vi "Front Panel Clean-Up.vi"(6 "Variant in":variant, 7 "Shift Pressed?":bool, 8 "error in (no error)":errorcluster, 10 "QD Combo Box Ref":refnum<vi>, 11 "QD Launch VI Ref":refnum<vi>) -> (0 "error out":errorcluster, 4 "Variant out":variant)   [LabVIEW 2011, in "LVH-Toolbox.lvlib"]
doc: "Write a 1-2 sentence description of the functionality of your plugin here. Replace the \"$\" below with the character you wish to assign as the default shortcut for this plugin. Do not add any text after the 'Default Shortcut' line below.\n\nDefault Shortcut - [$]"
uses:
  <vilib>/LabVIEW Hacker/LVH-Toolbox/LVH-Toolbox.lvlib
panel:
  in  "Undo Name":string="Quick Drop Front Panel Clean-Up"
  # "Do not change the connector pane of this VI.\n\nSee the block diagram for directions on how to use this template."
  # "Specify the name of the Undo transaction"
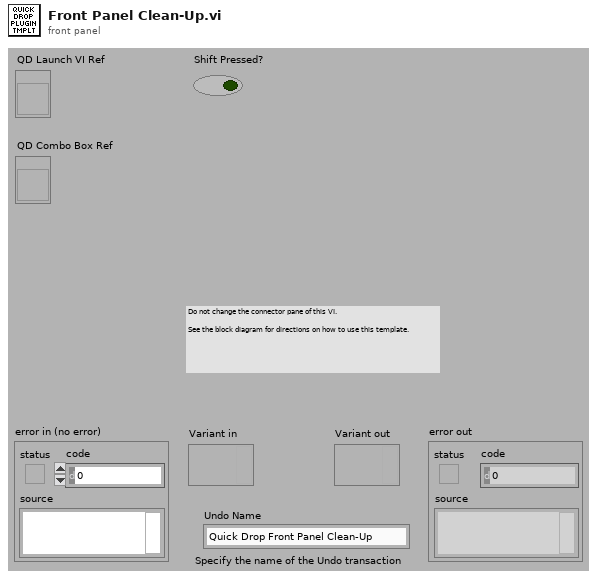
[diagram p1: front panel]
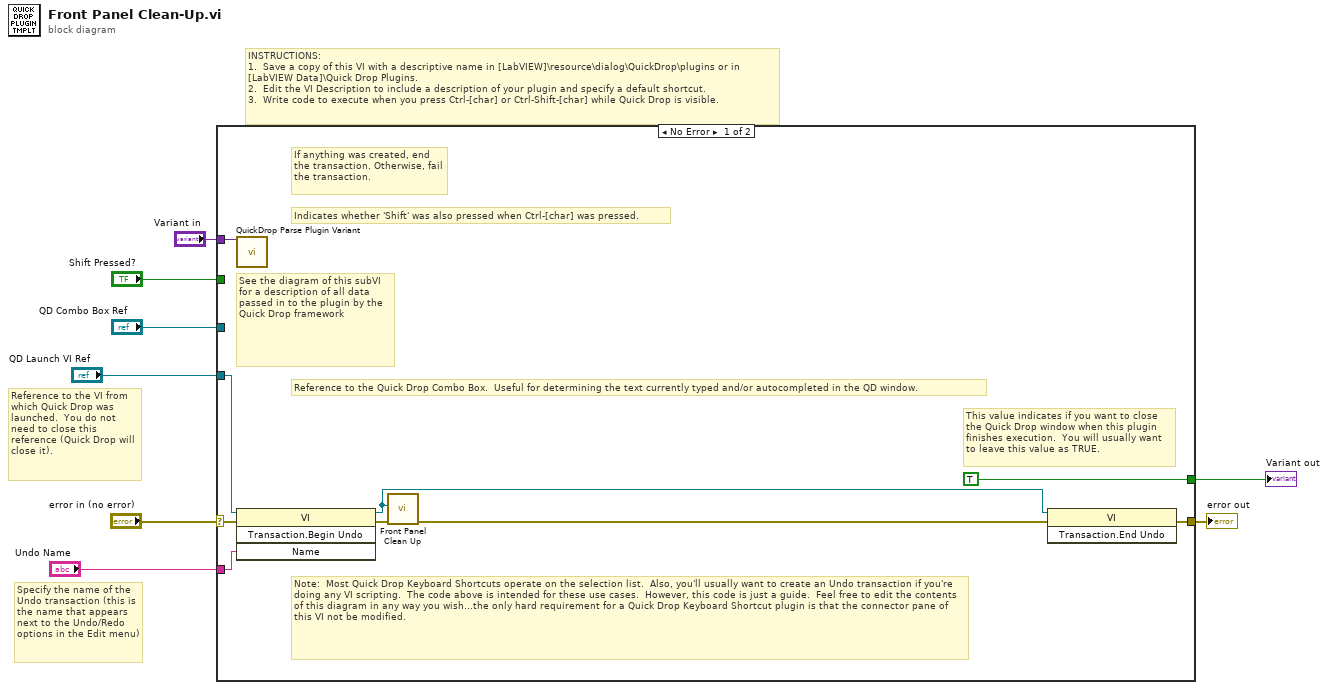
[diagram p0: block diagram]
diagram:
  # "Specify the name of the Undo transaction (this is the name that appears next to the Undo/Redo options in the Edit menu)"
  # "Reference to the VI from which Quick Drop was launched.  You do not need to close this reference (Quick Drop will close it)."
  # "INSTRUCTIONS:\n1.  Save a copy of this VI with a descriptive name in [LabVIEW]\\resource\\dialog\\QuickDrop\\plugins or in [LabVIEW Data]\\Quick Drop Plugins.\n2.  Edit the VI Description to include a description of your plugin and specify a default shortcut. \n3.  Write code to execute when you press Ctrl-[char] or Ctrl-Shift-[char] while Quick Drop is visible."
  n1 = case shown="No Error" "error in (no error)" {
    selector: "error in (no error)" -> [w16 w18]
    tunnel: [w12 w18] -> w7
    tunnel: "QD Launch VI Ref" -> [w15 _]
    tunnel: "Shift Pressed?" -> [_ _]
    tunnel: "QD Combo Box Ref" -> [_ _]
    tunnel: "Variant in" -> [w17 _]
    tunnel: "Undo Name" -> [w14 _]
    tunnel: [TRUE _] -> w1
    frame No Error {
      # "Note:  Most Quick Drop Keyboard Shortcuts operate on the selection list.  Also, you'll usually want to create an Undo transaction if you're doing any VI scripting.  The code above is intended for these use cases.  However, this code is just a guide.  Feel free to edit the contents of this diagram in any way you wish...the only hard requirement for a Quick Drop Keyboard Shortcut plugin is that the connector pane of this VI not be modified."
      # "If anything was created, end the transaction. Otherwise, fail the transaction."
      # "This value indicates if you want to close the Quick Drop window when this plugin finishes execution.  You will usually want to leave this value as TRUE."
      # "See the diagram of this subVI for a description of all data passed in to the plugin by the Quick Drop framework"
      # "Reference to the Quick Drop Combo Box.  Useful for determining the text currently typed and/or autocompleted in the QD window."
      # "Indicates whether 'Shift' was also pressed when Ctrl-[char] was pressed."
      n2 = call <vilib>:"QuickDrop Parse Plugin Variant.vi"("QDKS Variant in"=w17) -> ()  [unwired: 12 in, 3 out]
      n3 = invoke class="VI" method="Transaction.Begin Undo"(reference=w15, error in=w16, "Name"=w14) -> (reference out=w11:refnum<vi>, error out=w10:errorcluster)  [unwired: 1 in, 2 out]
      n4 = call <vilib>:"Front Panel Clean Up.vi"("Error In"=w10, "VI Ref"=w11) -> ("Error Out"=w9:errorcluster)  [unwired: 9 in]
      n5 = invoke class="VI" method="Transaction.End Undo"(reference=w11, error in=w9) -> (error out=w12:errorcluster)  [unwired: 1 in, 2 out]
    }
    frame Error {
    }
  }
  "error out" <- w7
  "Variant out" <- w1
